vi "GetSampleCount.vi"(4 "error in (no error)":errorcluster, 6 "Device Key In":string, 7 "PM Cmds In":refnum<k24>) -> (0 "error out":errorcluster, 1 "Sample Count":string, 2 "Device Key Out":string, 3 "PM Cmds Out":refnum<k24>)   [LabVIEW 2009]
uses:
  C:/Code/Apps/Utilities/PM2935/PMWinApp/PM_Installer/Master/Samples/LabVIEWSample/LabVIEW 2009/PowerMeterCommands.dll
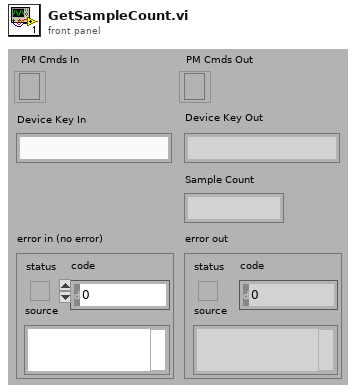
[diagram p1: front panel]
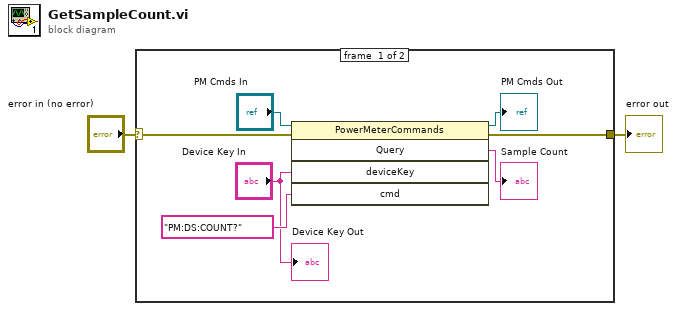
[diagram p0: block diagram]
diagram:
  n1 = case shown="No Error" "error in (no error)" {
    selector: "error in (no error)" -> [w9 w10]
    tunnel: [w8 w10] -> w1
    frame #0 {
      n2 = invoke class="PowerMeterCommands" method="Query"(reference="PM Cmds In", error in=w9, "deviceKey"="Device Key In", "cmd"="PM:DS:COUNT?") -> (reference out=→"PM Cmds Out":refnum<k24>, error out=w8:errorcluster, "Query"=→"Sample Count":string)  [unwired: 1 in, 2 out]
      "Device Key Out" <- "Device Key In"
    }
    frame #1 {
    }
  }
  "error out" <- w1
